vi "FPGA Set Defaults.vi"(8 "error in (no error)":errorcluster) -> (0 "error out":errorcluster)   [LabVIEW 2017]
doc: "Sets the default configuration of the FPGA."
uses:
  FPGA Global Variables.vi
  <vilib>/Utility/error.llb/Error Cluster From Error Code.vi
  <vilib>/rvi/errors/niLvFpgaAdjustHostInterfaceError.vi
  <vilib>/rvi/interface/nirviReadWriteControl/nirviReadWriteControl.xnode
  NiFpgaLv.dll
  <vilib>/rvi/interface/Simulation/niFpgaSimulationCallBeginRW.vi
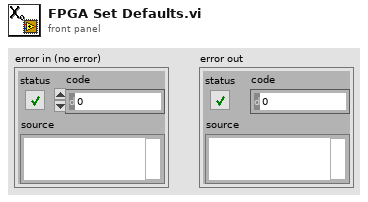
[diagram p1: front panel]
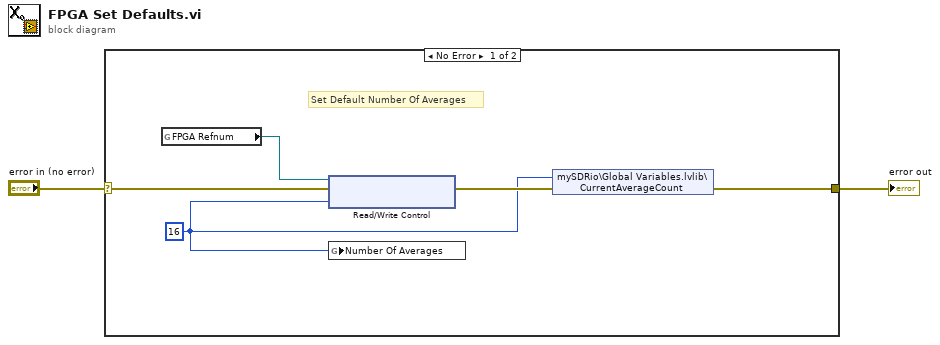
[diagram p0: block diagram]
diagram:
  n1 = case shown="No Error" "error in (no error)" {
    selector: "error in (no error)" -> [w6 w8]
    tunnel: [w4 w8] -> w2
    frame No Error {
      w3 = u32 16 ("Number Of Averages")
      # "Set Default Number Of Averages"
      n2 = global read "FPGA Global Variables.vi" "FPGA Refnum"() -> (w7:refnum<k20>)
      n3 = xnode "Read/Write Control"("FPGA VI Reference In"=w7, "error in"=w6, "Windows in Average"=w3) -> ("error out"=w5:errorcluster)  [unwired: 1 out]
      n4 = global write "FPGA Global Variables.vi" "Number Of Averages"(w3) -> ()
      n5 = shared-variable "mySDRio\\Global Variables.lvlib\\CurrentAverageCount"(w3, error in=w5) -> (error out=w4:errorcluster)
    }
    frame Error {
    }
  }
  "error out" <- w2
